vi "KickValueTestMeanAndStd.vi"(8 "error in (no error)":errorcluster, 9 "ResultKickForce2DArray":dbl[][](array[numeric])=[[-4.0, 40.0, 0.0, 0.0, 0.0, 0.0], [-4.0, 50.0, 1.0, 0.0, 0.0, 4.1076070568751994], [-4.0, 60.0, 2.0, 0.0, 0.0, 4.095926992624832], [-4.0, 70.0, 3.0, 0.0, 0.0, 2.769868919049422], [-3.0, 40.0, 0.0, 1.0, 0.0, 2.6076315632093388], [-3.0, 50.0, 1.0, 1.0, 0.0, 3.9530709630255614], [-3.0, 60.0, 2.0, 1.0, 0.0, 3.9355536131771096], [-3.0, 70.0, 3.0, 1.0, 0.0, 3.9413927297932605], [-2.0, 40.0, 0.0, 2.0, 0.0, 2.5712986717028237], [-2.0, 50.0, 1.0, 2.0, 0.0, 3.5375543710104185], [-2.0, 60.0, 2.0, 2.0, 0.0, 3.7985367001939907], [-2.0, 70.0, 3.0, 2.0, 0.0, 2.7618728631501654], [-1.0, 40.0, 0.0, 3.0, 0.0, 2.3441865147254464], [-1.0, 50.0, 1.0, 3.0, 0.0, 3.440702670348366], [-1.0, 60.0, 2.0, 3.0, 0.0, 3.446543617982584], [-1.0, 70.0, 3.0, 3.0, 0.0, 2.5507802832423083], [0.0, 40.0, 0.0, 4.0, 0.0, 3.0332425578286957], [0.0, 50.0, 1.0, 4.0, 0.0, 2.7845060774782424], [0.0, 60.0, 2.0, 4.0, 0.0, 3.296275627247479], [0.0, 70.0, 3.0, 4.0, 0.0, 2.770205826373778], [1.0, 40.0, 0.0, 5.0, 0.0, 2.596597848336675], [1.0, 50.0, 1.0, 5.0, 0.0, 3.220303025605171], [1.0, 60.0, 2.0, 5.0, 0.0, 3.1568069810724424], [1.0, 70.0, 3.0, 5.0, 0.0, 2.800139309735594], [2.0, 40.0, 0.0, 6.0, 0.0, 2.6720998783357253], [2.0, 50.0, 1.0, 6.0, 0.0, 3.139218221519372], [2.0, 60.0, 2.0, 6.0, 0.0, 3.6201424409293503], [2.0, 70.0, 3.0, 6.0, 0.0, 3.1508964547516727], [-4.0, 40.0, 0.0, 0.0, 1.0, 3.862091337304868], [-4.0, 50.0, 1.0, 0.0, 1.0, 0.0], [-4.0, 60.0, 2.0, 0.0, 1.0, 2.7702973772771355], [-4.0, 70.0, 3.0, 0.0, 1.0, 4.101766109240982], [-3.0, 40.0, 0.0, 1.0, 1.0, 3.7367526575540504], [-3.0, 50.0, 1.0, 1.0, 1.0, 3.9355536131771096], [-3.0, 60.0, 2.0, 1.0, 1.0, 2.8454606689337623], [-3.0, 70.0, 3.0, 1.0, 1.0, 2.9486733263611047], [-2.0, 40.0, 0.0, 2.0, 1.0, 3.5530191496055923], [-2.0, 50.0, 1.0, 2.0, 1.0, 2.7793938750347515], [-2.0, 60.0, 2.0, 2.0, 1.0, 2.773747015315652], [-2.0, 70.0, 3.0, 2.0, 1.0, 2.785425248547953], [-1.0, 40.0, 0.0, 3.0, 1.0, 2.358036335385391], [-1.0, 50.0, 1.0, 3.0, 1.0, 3.444870067469206], [-1.0, 60.0, 2.0, 3.0, 1.0, 2.544942997644225], [-1.0, 70.0, 3.0, 3.0, 1.0, 2.577807940931552], [0.0, 40.0, 0.0, 4.0, 1.0, 2.6088272180071894], [0.0, 50.0, 1.0, 4.0, 1.0, 2.7994032404725986], [0.0, 60.0, 2.0, 4.0, 1.0, 3.3555676542980244], [0.0, 70.0, 3.0, 4.0, 1.0, 3.3439040692102604], [1.0, 40.0, 0.0, 5.0, 1.0, 2.6087320050676976], [1.0, 50.0, 1.0, 5.0, 1.0, 2.823495776200196], [1.0, 60.0, 2.0, 5.0, 1.0, 2.823495776200196], [1.0, 70.0, 3.0, 5.0, 1.0, 2.817654828565978], [2.0, 40.0, 0.0, 6.0, 1.0, 2.752800168627423], [2.0, 50.0, 1.0, 6.0, 1.0, 2.9375389054947476], [2.0, 60.0, 2.0, 6.0, 1.0, 3.113708477807797], [2.0, 70.0, 3.0, 6.0, 1.0, 2.937542567530882], [-4.0, 40.0, 0.0, 0.0, 2.0, 2.5680467836155603], [-4.0, 50.0, 1.0, 0.0, 2.0, 0.0], [-4.0, 60.0, 2.0, 0.0, 2.0, 2.7527818584467507], [-4.0, 70.0, 3.0, 0.0, 2.0, 4.090091538044815], [-3.0, 40.0, 0.0, 1.0, 2.0, 2.4683588359674875], [-3.0, 50.0, 1.0, 1.0, 2.0, 0.0], [-3.0, 60.0, 2.0, 1.0, 2.0, 3.9530727940436288], [-3.0, 70.0, 3.0, 1.0, 2.0, 0.0], [-2.0, 40.0, 0.0, 2.0, 2.0, 2.5712986717028237], [-2.0, 50.0, 1.0, 2.0, 2.0, 3.801988169250574], [-2.0, 60.0, 2.0, 2.0, 2.0, 2.705407927995304], [-2.0, 70.0, 3.0, 2.0, 2.0, 2.785232991650902], [-1.0, 40.0, 0.0, 3.0, 2.0, 2.3580381664034578], [-1.0, 50.0, 1.0, 3.0, 2.0, 3.458221851214885], [-1.0, 60.0, 2.0, 3.0, 2.0, 2.5602905910831004], [-1.0, 70.0, 3.0, 3.0, 2.0, 2.5486086958146648], [0.0, 40.0, 0.0, 4.0, 2.0, 2.591309868158738], [0.0, 50.0, 1.0, 4.0, 2.0, 2.8110814737048995], [0.0, 60.0, 2.0, 4.0, 2.0, 2.79034702511246], [0.0, 70.0, 3.0, 4.0, 2.0, 2.784507908496309], [1.0, 40.0, 0.0, 5.0, 2.0, 3.30352279675727], [1.0, 50.0, 1.0, 5.0, 2.0, 2.8351758404505643], [1.0, 60.0, 2.0, 5.0, 2.0, 2.805141651095055], [1.0, 70.0, 3.0, 5.0, 2.0, 3.1626515907427946], [2.0, 40.0, 0.0, 6.0, 2.0, 2.6920762854483637], [2.0, 50.0, 1.0, 6.0, 2.0, 2.8651312960291864], [2.0, 60.0, 2.0, 6.0, 2.0, 3.631820674161651], [2.0, 70.0, 3.0, 6.0, 2.0, 2.8826816042028467], [-4.0, 40.0, 0.0, 0.0, 3.0, 0.0], [-4.0, 50.0, 1.0, 0.0, 3.0, 0.0], [-4.0, 60.0, 2.0, 0.0, 3.0, 3.5612129554561016], [-4.0, 70.0, 3.0, 0.0, 3.0, 2.7586191440448347], [-3.0, 40.0, 0.0, 1.0, 3.0, 2.578977961476463], [-3.0, 50.0, 1.0, 1.0, 3.0, 3.970588312874013], [-3.0, 60.0, 2.0, 1.0, 3.0, 3.55085305523215], [-3.0, 70.0, 3.0, 1.0, 3.0, 2.745316797786969], [-2.0, 40.0, 0.0, 2.0, 3.0, 2.5890119404844607], [-2.0, 50.0, 1.0, 2.0, 3.0, 2.767711979766316], [-2.0, 60.0, 2.0, 2.0, 3.0, 2.7735529274005337], [-2.0, 70.0, 3.0, 2.0, 3.0, 2.8029407673783377], [-1.0, 40.0, 0.0, 3.0, 3.0, 2.7240074095214433], [-1.0, 50.0, 1.0, 3.0, 3.0, 2.5771414503551084], [-1.0, 60.0, 2.0, 3.0, 3.0, 2.575638184521976], [-1.0, 70.0, 3.0, 3.0, 3.0, 2.5661297076992513], [0.0, 40.0, 0.0, 4.0, 3.0, 3.1217466471225985], [0.0, 50.0, 1.0, 4.0, 3.0, 2.8227597069372004], [0.0, 60.0, 2.0, 4.0, 3.0, 2.811085135741034], [0.0, 70.0, 3.0, 4.0, 3.0, 2.834439771187569], [1.0, 40.0, 0.0, 5.0, 3.0, 2.63594093354559], [1.0, 50.0, 1.0, 5.0, 3.0, 2.810528506248619], [1.0, 60.0, 2.0, 5.0, 3.0, 2.828992492437789], [1.0, 70.0, 3.0, 5.0, 3.0, 2.8280495181332053], [2.0, 40.0, 0.0, 6.0, 3.0, 2.776035787899593], [2.0, 50.0, 1.0, 6.0, 3.0, 2.9762978959402404], [2.0, 60.0, 2.0, 6.0, 3.0, 2.9352373157843368], [2.0, 70.0, 3.0, 6.0, 3.0, 2.8592921794130355], [-4.0, 40.0, 0.0, 0.0, 4.0, 2.5563722124193933], [-4.0, 50.0, 1.0, 0.0, 4.0, 2.760913409682977], [-4.0, 60.0, 2.0, 0.0, 4.0, 2.735262677580232], [-4.0, 70.0, 3.0, 0.0, 4.0, 4.1076052258571325], [-3.0, 40.0, 0.0, 1.0, 4.0, 3.719238969741733], [-3.0, 50.0, 1.0, 1.0, 4.0, 3.9997857269728336], [-3.0, 60.0, 2.0, 1.0, 4.0, 2.76954849088767], [-3.0, 70.0, 3.0, 1.0, 4.0, 0.0], [-2.0, 40.0, 0.0, 2.0, 4.0, 3.5681488518944766], [-2.0, 50.0, 1.0, 2.0, 4.0, 2.8027466794632194], [-2.0, 60.0, 2.0, 2.0, 4.0, 2.767711979766316], [-2.0, 70.0, 3.0, 2.0, 4.0, 2.773747015315652], [-1.0, 40.0, 0.0, 3.0, 4.0, 2.3543669751788165], [-1.0, 50.0, 1.0, 3.0, 4.0, 2.5814773011381265], [-1.0, 60.0, 2.0, 3.0, 4.0, 2.577807940931552], [-1.0, 70.0, 3.0, 3.0, 4.0, 2.577807940931552], [0.0, 40.0, 0.0, 4.0, 4.0, 2.626348229891776], [0.0, 50.0, 1.0, 4.0, 4.0, 2.7994032404725986], [0.0, 60.0, 2.0, 4.0, 4.0, 2.796200789873148], [0.0, 70.0, 3.0, 4.0, 4.0, 2.8110814737048995], [1.0, 40.0, 0.0, 5.0, 4.0, 2.615404234904403], [1.0, 50.0, 1.0, 5.0, 4.0, 2.81147331157127], [1.0, 60.0, 2.0, 5.0, 4.0, 3.1392914622420576], [1.0, 70.0, 3.0, 5.0, 4.0, 2.799306196515039], [2.0, 40.0, 0.0, 6.0, 4.0, 2.6745534425457103], [2.0, 50.0, 1.0, 6.0, 4.0, 3.125119382402294], [2.0, 60.0, 2.0, 6.0, 4.0, 2.855313377153112], [2.0, 70.0, 3.0, 6.0, 4.0, 2.956563183212466], [-4.0, 40.0, 0.0, 0.0, 5.0, 2.5731498309687155], [-4.0, 50.0, 1.0, 0.0, 5.0, 3.5442192767748555], [-4.0, 60.0, 2.0, 0.0, 5.0, 0.0], [-4.0, 70.0, 3.0, 0.0, 5.0, 0.0], [-3.0, 40.0, 0.0, 1.0, 5.0, 3.725074424321749], [-3.0, 50.0, 1.0, 1.0, 5.0, 3.96475102727593], [-3.0, 60.0, 2.0, 1.0, 5.0, 2.7569950310192697], [-3.0, 70.0, 3.0, 1.0, 5.0, 3.9647491962578627], [-2.0, 40.0, 0.0, 2.0, 5.0, 3.362320448929684], [-2.0, 50.0, 1.0, 2.0, 5.0, 2.7638009251748774], [-2.0, 60.0, 2.0, 2.0, 5.0, 3.810216764444359], [-2.0, 70.0, 3.0, 2.0, 5.0, 2.785425248547953], [-1.0, 40.0, 0.0, 3.0, 5.0, 2.369716399635759], [-1.0, 50.0, 1.0, 3.0, 5.0, 2.5661297076992513], [-1.0, 60.0, 2.0, 3.0, 5.0, 3.440702670348366], [-1.0, 70.0, 3.0, 3.0, 5.0, 2.5581208346735242], [0.0, 40.0, 0.0, 4.0, 5.0, 2.6088272180071894], [0.0, 50.0, 1.0, 4.0, 5.0, 2.8110814737048995], [0.0, 60.0, 2.0, 4.0, 5.0, 3.3731014833090804], [0.0, 70.0, 3.0, 4.0, 5.0, 2.7994032404725986], [1.0, 40.0, 0.0, 5.0, 5.0, 2.6145692906657816], [1.0, 50.0, 1.0, 5.0, 5.0, 3.5665540351579867], [1.0, 60.0, 2.0, 5.0, 5.0, 2.810528506248619], [1.0, 70.0, 3.0, 5.0, 5.0, 3.231992244945875], [2.0, 40.0, 0.0, 6.0, 5.0, 3.386310447645522], [2.0, 50.0, 1.0, 6.0, 5.0, 2.870970412645337], [2.0, 60.0, 2.0, 6.0, 5.0, 2.9550580863612668], [2.0, 70.0, 3.0, 6.0, 5.0, 2.865164254354395], [-4.0, 40.0, 0.0, 0.0, 6.0, 0.0], [-4.0, 50.0, 1.0, 0.0, 6.0, 2.764456429642918], [-4.0, 60.0, 2.0, 0.0, 6.0, 2.793655674759805], [-4.0, 70.0, 3.0, 0.0, 6.0, 0.0], [-3.0, 40.0, 0.0, 1.0, 6.0, 0.0], [-3.0, 50.0, 1.0, 1.0, 6.0, 0.0], [-3.0, 60.0, 2.0, 1.0, 6.0, 0.0], [-3.0, 70.0, 3.0, 1.0, 6.0, 0.0], [-2.0, 40.0, 0.0, 2.0, 6.0, 2.508994619931812], [-2.0, 50.0, 1.0, 2.0, 6.0, 2.7170861612276047], [-2.0, 60.0, 2.0, 2.0, 6.0, 2.8496537003075426], [-2.0, 70.0, 3.0, 2.0, 6.0, 2.796909393865136], [-1.0, 40.0, 0.0, 3.0, 6.0, 2.3807281422916167], [-1.0, 50.0, 1.0, 3.0, 6.0, 2.548612357850799], [-1.0, 60.0, 2.0, 3.0, 6.0, 2.5661297076992513], [-1.0, 70.0, 3.0, 3.0, 6.0, 3.440702670348366], [0.0, 40.0, 0.0, 4.0, 6.0, 2.6088272180071894], [0.0, 50.0, 1.0, 4.0, 6.0, 2.8227597069372004], [0.0, 60.0, 2.0, 4.0, 6.0, 2.8110814737048995], [0.0, 70.0, 3.0, 4.0, 6.0, 2.7961843107105433], [1.0, 40.0, 0.0, 5.0, 6.0, 2.6245721423666373], [1.0, 50.0, 1.0, 5.0, 6.0, 3.2080992901875964], [1.0, 60.0, 2.0, 5.0, 6.0, 2.9029912566037064], [1.0, 70.0, 3.0, 5.0, 6.0, 3.156561624651444], [2.0, 40.0, 0.0, 6.0, 6.0, 2.688441714585065], [2.0, 50.0, 1.0, 6.0, 6.0, 2.8768095292614873], [2.0, 60.0, 2.0, 6.0, 6.0, 2.88480192312461], [2.0, 70.0, 3.0, 6.0, 6.0, 2.943376191092831], [-4.0, 40.0, 0.0, 0.0, 7.0, 3.8737714015552367], [-4.0, 50.0, 1.0, 0.0, 7.0, 0.0], [-4.0, 60.0, 2.0, 0.0, 7.0, 2.7702973772771355], [-4.0, 70.0, 3.0, 0.0, 7.0, 2.7695613080141404], [-3.0, 40.0, 0.0, 1.0, 7.0, 3.7192353077055986], [-3.0, 50.0, 1.0, 1.0, 7.0, 2.7686750952696384], [-3.0, 60.0, 2.0, 1.0, 7.0, 0.0], [-3.0, 70.0, 3.0, 1.0, 7.0, 0.0], [-2.0, 40.0, 0.0, 2.0, 7.0, 2.6006920047348294], [-2.0, 50.0, 1.0, 2.0, 7.0, 3.5669586901508272], [-2.0, 60.0, 2.0, 2.0, 7.0, 3.572799637785045], [-2.0, 70.0, 3.0, 2.0, 7.0, 2.796909393865136], [-1.0, 40.0, 0.0, 3.0, 7.0, 2.3813946328680604], [-1.0, 50.0, 1.0, 3.0, 7.0, 2.5581208346735242], [-1.0, 60.0, 2.0, 3.0, 7.0, 2.554447812430815], [-1.0, 70.0, 3.0, 3.0, 7.0, 3.440702670348366], [0.0, 40.0, 0.0, 4.0, 7.0, 3.115907530506448], [0.0, 50.0, 1.0, 4.0, 7.0, 2.816918759302983], [0.0, 60.0, 2.0, 4.0, 7.0, 2.8110814737048995], [0.0, 70.0, 3.0, 4.0, 7.0, 3.361421419058712], [1.0, 40.0, 0.0, 5.0, 7.0, 2.6329197537347877], [1.0, 50.0, 1.0, 5.0, 7.0, 2.834340896211943], [1.0, 60.0, 2.0, 5.0, 7.0, 3.566557697194121], [1.0, 70.0, 3.0, 5.0, 7.0, 2.828992492437789], [2.0, 40.0, 0.0, 6.0, 7.0, 3.386310447645522], [2.0, 50.0, 1.0, 6.0, 7.0, 2.888520720818997], [2.0, 60.0, 2.0, 6.0, 7.0, 2.9528901609697575], [2.0, 70.0, 3.0, 6.0, 7.0, 3.1020339066116303], [-4.0, 40.0, 0.0, 0.0, 8.0, 2.567310714352565], [-4.0, 50.0, 1.0, 0.0, 8.0, 4.1192852901075], [-4.0, 60.0, 2.0, 0.0, 8.0, 0.0], [-4.0, 70.0, 3.0, 0.0, 8.0, 2.6537164569415106], [-3.0, 40.0, 0.0, 1.0, 8.0, 0.0], [-3.0, 50.0, 1.0, 1.0, 8.0, 2.763713036307654], [-3.0, 60.0, 2.0, 1.0, 8.0, 0.0], [-3.0, 70.0, 3.0, 1.0, 8.0, 3.5485752687566117], [-2.0, 40.0, 0.0, 2.0, 8.0, 2.5773318762340924], [-2.0, 50.0, 1.0, 2.0, 8.0, 2.785425248547953], [-2.0, 60.0, 2.0, 2.0, 8.0, 3.5786405854192624], [-2.0, 70.0, 3.0, 2.0, 8.0, 3.584270965975758], [-1.0, 40.0, 0.0, 3.0, 8.0, 2.3638736209834743], [-1.0, 50.0, 1.0, 3.0, 8.0, 3.4523827345987343], [-1.0, 60.0, 2.0, 3.0, 8.0, 2.552281718057374], [-1.0, 70.0, 3.0, 3.0, 8.0, 2.5719688243154017], [0.0, 40.0, 0.0, 4.0, 8.0, 2.6114492358793524], [0.0, 50.0, 1.0, 4.0, 8.0, 2.8811563661529083], [0.0, 60.0, 2.0, 4.0, 8.0, 2.799416057599068], [0.0, 70.0, 3.0, 4.0, 8.0, 2.834441602205636], [1.0, 40.0, 0.0, 5.0, 8.0, 2.6212415205024864], [1.0, 50.0, 1.0, 5.0, 8.0, 2.8056341949551196], [1.0, 60.0, 2.0, 5.0, 8.0, 2.8289943234558566], [1.0, 70.0, 3.0, 5.0, 8.0, 2.823495776200196], [2.0, 40.0, 0.0, 6.0, 8.0, 2.65335025332808], [2.0, 50.0, 1.0, 6.0, 8.0, 2.8768095292614873], [2.0, 60.0, 2.0, 6.0, 8.0, 3.1251157203661597], [2.0, 70.0, 3.0, 6.0, 8.0, 2.97624662743436], [-4.0, 40.0, 0.0, 0.0, 9.0, 2.591410574152431], [-4.0, 50.0, 1.0, 0.0, 9.0, 4.1192852901075], [-4.0, 60.0, 2.0, 0.0, 9.0, 4.119287121125568], [-4.0, 70.0, 3.0, 0.0, 9.0, 4.13096535435787], [-3.0, 40.0, 0.0, 1.0, 9.0, 3.742589943152134], [-3.0, 50.0, 1.0, 1.0, 9.0, 2.786670340833617], [-3.0, 60.0, 2.0, 1.0, 9.0, 3.976429260508231], [-3.0, 70.0, 3.0, 1.0, 9.0, 2.8679455707984003], [-2.0, 40.0, 0.0, 2.0, 9.0, 2.518371263453702], [-2.0, 50.0, 1.0, 2.0, 9.0, 2.693729694763003], [-2.0, 60.0, 2.0, 2.0, 9.0, 2.796909393865136], [-2.0, 70.0, 3.0, 2.0, 9.0, 2.8087817150125556], [-1.0, 40.0, 0.0, 3.0, 9.0, 2.369716399635759], [-1.0, 50.0, 1.0, 3.0, 9.0, 2.601164407396155], [-1.0, 60.0, 2.0, 3.0, 9.0, 2.5661297076992513], [-1.0, 70.0, 3.0, 3.0, 9.0, 3.446543617982584], [0.0, 40.0, 0.0, 4.0, 9.0, 2.63802463210601], [0.0, 50.0, 1.0, 4.0, 9.0, 2.834450757295972], [0.0, 60.0, 2.0, 4.0, 9.0, 2.8286116406798216], [0.0, 70.0, 3.0, 4.0, 9.0, 2.79034702511246], [1.0, 40.0, 0.0, 5.0, 9.0, 2.626251185934217], [1.0, 50.0, 1.0, 5.0, 9.0, 3.156814305144711], [1.0, 60.0, 2.0, 5.0, 9.0, 2.828082476458414], [1.0, 70.0, 3.0, 5.0, 9.0, 2.823155206839706], [2.0, 40.0, 0.0, 6.0, 9.0, 2.7564731908701314], [2.0, 50.0, 1.0, 6.0, 9.0, 2.9375389054947476], [2.0, 60.0, 2.0, 6.0, 9.0, 2.894326879109939], [2.0, 70.0, 3.0, 6.0, 9.0, 3.160227322821884]], 10 "Sample":dbl=1.0) -> (0 "error out":errorcluster, 2 "KickForceMean":T1=[[-4.0, 50.0, 3.274877129436019], [-4.0, 60.0, 4.143627251185135], [-4.0, 70.0, 2.701105442430398], [-4.0, 80.0, 2.899398392263049], [-4.0, 90.0, 2.7566434755503764], [-4.0, 100.0, 3.1909487542919313], [-3.0, 50.0, 3.3639282862390965], [-3.0, 60.0, 2.9052336433966133], [-3.0, 70.0, 3.3737278949344987], [-3.0, 80.0, 3.4555239478161606], [-3.0, 90.0, 3.4188584213607798], [-3.0, 100.0, 3.29704648585375], [-2.0, 50.0, 3.4168797011695435], [-2.0, 60.0, 3.5979584363670813], [-2.0, 70.0, 3.5810410501053007], [-2.0, 80.0, 3.3547691269742943], [-2.0, 90.0, 3.368842331838431], [-2.0, 100.0, 3.3547302687019798], [-1.0, 50.0, 3.3574503477639617], [-1.0, 60.0, 3.3417640159826627], [-1.0, 70.0, 3.04407567449978], [-1.0, 80.0, 3.2440153199141566], [-1.0, 90.0, 3.2448856638354098], [-1.0, 100.0, 3.3577211349914475], [0.0, 50.0, 3.3567610711849043], [0.0, 60.0, 3.3393019070216976], [0.0, 70.0, 3.354224093929638], [0.0, 80.0, 3.3697374962268167], [0.0, 90.0, 3.4324429478474396], [0.0, 100.0, 3.3490341749415196], [1.0, 50.0, 3.513340784643937], [1.0, 60.0, 3.46354055180706], [1.0, 70.0, 3.4204188556468975], [1.0, 80.0, 3.593593696187893], [1.0, 90.0, 3.54274876582048], [1.0, 100.0, 3.4868431049619075], [2.0, 50.0, 3.5850540313691437], [2.0, 60.0, 3.5291864149970777], [2.0, 70.0, 3.669538222219838], [2.0, 80.0, 3.5181089591372543], [2.0, 90.0, 3.6555360201674154], [2.0, 100.0, 3.651149714664325]])   [LabVIEW 2021, in "Game.lvclass"]
uses:
  Game.lvclass
  Kickmeanvalues.ctl
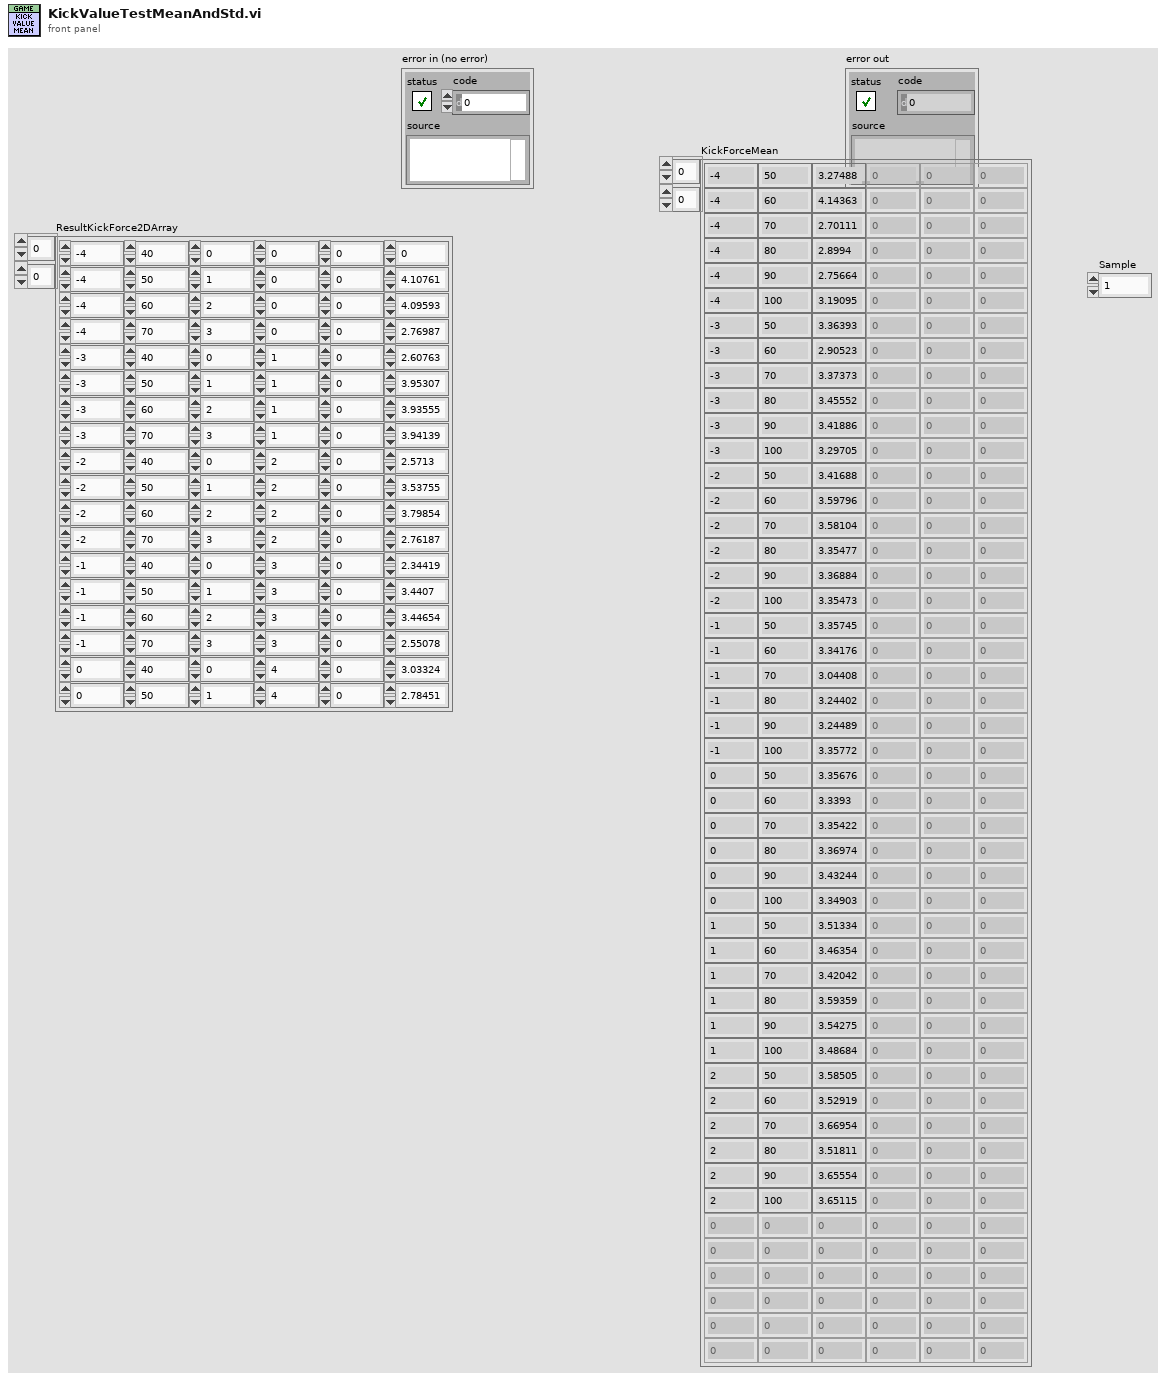
[diagram p1: front panel]
types:
  T1 = typedef "Kickmeanvalues.ctl" = dbl[][]
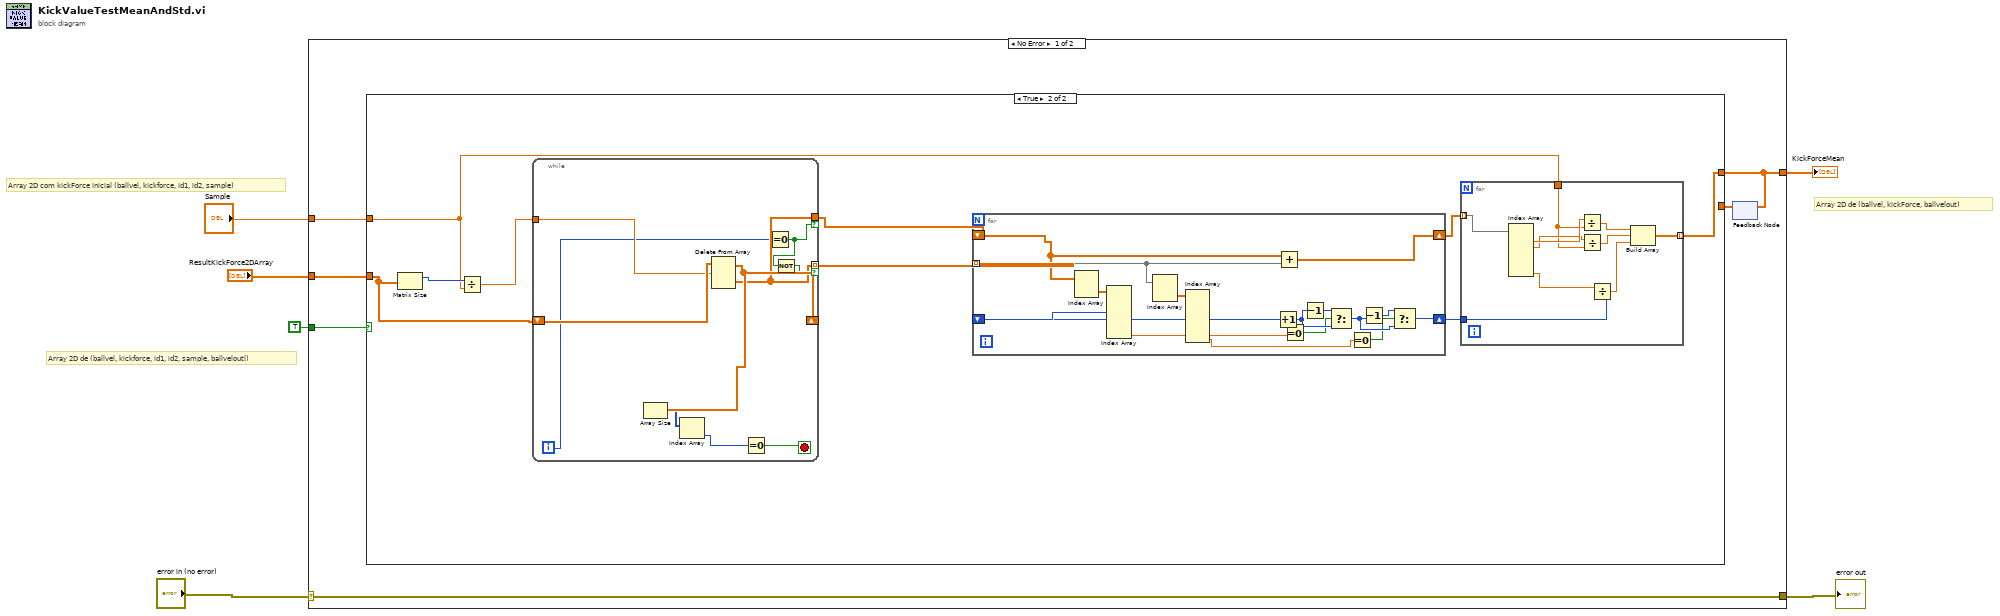
[diagram p0: block diagram]
diagram:
  # "Array 2D de (ballvel, kickForce, ballvelout)"
  # "Array 2D com kickForce inicial (ballvel, kickforce, id1, id2, sample)"
  # "Array 2D de (ballvel, kickforce, id1, id2, sample, ballveloutl)"
  n1 = case shown="No Error" "error in (no error)" {
    selector: "error in (no error)" -> [w12 w59]
    tunnel: [w12 w59] -> w4
    tunnel: "ResultKickForce2DArray" -> [w11 _]
    tunnel: [w10 _] -> w1
    tunnel: TRUE ("firstCall") -> [w8 _]
    tunnel: "Sample" -> [w7 _]
    frame No Error {
      n2 = feedback #1() -> (w9:dbl[][])  [unwired: 1 in]
      n3 = case shown="True" w8 {
        tunnel: w11 -> [_ w17]
        tunnel: [w13 w15] -> w10
        tunnel: w9 -> [w13 _]
        tunnel: w7 -> [_ w14]
        frame False {
        }
        frame True {
          n4 = Matrix Size(0:w17) -> (1:w23:i32)  [unwired: 1 out]
          n5 = Divide(x=w23, y=w14) -> (x/y=w22:dbl)
          n6 = while {
            tunnel: w22 -> [w57]
            tunnel: [w52] -> w21 mode=indexing if=w49
            shift-right: [w56] -> _
            shift-left: w17 -> [w58]
            tunnel: [w52] -> w18 if=w50
            i -> [w51]
            stop <- w53 stop-if-true
            n7 = Delete From Array(array=w58, length=w57) -> (deleted portion=w52:dbl[][], array with subset deleted=w56:dbl[][])  [unwired: 2 in]
            n8 = Array Size(array=w56) -> (size(s)=w55:i32[])
            n9 = Index Array(array=w55) -> (element=w54:i32)  [unwired: 1 in]
            n10 = Equal To 0?(x=w54) -> (x = 0?=w53:bool)
            n11 = Equal To 0?(x=w51) -> (x = 0?=w50:bool)
            n12 = Not(x=w50) -> (.not. x?=w49:bool)
          }
          n13 = for {
            shift-right: [w48] -> w16
            shift-left: w18 -> [w46]
            tunnel: w21 -> [w40] mode=indexing
            shift-right: [w34] -> w19
            shift-left: 1 -> [w47]
            n14 = Index Array(array=w46) -> (element=w45:dbl[])  [unwired: 2 in]
            n15 = Index Array(array=w45) -> (element #6=w42:dbl)  [unwired: 6 in, 5 out]
            n16 = Index Array(array=w40) -> (element=w39:dbl[])  [unwired: 2 in]
            n17 = Index Array(array=w39) -> (element #6=w36:dbl)  [unwired: 6 in, 5 out]
            n18 = Increment(x=w47) -> (x+1=w44:i32)
            n19 = Add(x=w46, y=w40) -> (x+y=w48:dbl[][])
            n20 = Equal To 0?(x=w42) -> (x = 0?=w41:bool)
            n21 = Decrement(x=w44) -> (x-1=w43:i32)
            n22 = Select(t=w43, s=w41, f=w44) -> (s? t:f=w37:i32)
            n23 = Equal To 0?(x=w36) -> (x = 0?=w35:bool)
            n24 = Decrement(x=w37) -> (x-1=w38:i32)
            n25 = Select(t=w38, s=w35, f=w37) -> (s? t:f=w34:i32)
          }
          n26 = for {
            tunnel: w19 -> [w33]
            tunnel: w16 -> [w28] mode=indexing
            tunnel: [w31] -> w15 mode=indexing
            tunnel: w14 -> [w24]
            n27 = Index Array(array=w28) -> (element #1=w27:dbl, element #2=w26:dbl, element #6=w25:dbl)  [unwired: 6 in, 3 out]
            n28 = Divide(x=w27, y=w24) -> (x/y=w30:dbl)
            n29 = Divide(x=w26, y=w24) -> (x/y=w29:dbl)
            n30 = Divide(x=w25, y=w33) -> (x/y=w32:dbl)
            n31 = Build Array(w30, w29, w32) -> (w31:dbl[])
          }
        }
      }
      n32 = feedback-in #1(w10) -> ()
    }
    frame Error {
    }
  }
  "error out" <- w4
  "KickForceMean" <- w1
